vi "rsscope_core_global.vi"() -> ()   [LabVIEW 2018] (continued)
 "Instrument Options"="", "Flags"=0, "Help"="The arithmetic mode defines how the final FFT result is calculated from the individual frame results.\n\nAvailable Repeated Capabilities:\nMath: M1, M2, M3, M4, M5, M6, M7, M8\r\n\nRemote-control command(s):\nCALCulate:MATH<m>:FFT:FRAMe:ARIThmetics"}, {"Level"=3, "Class Only"=FALSE, "Identifier"="RSSCOPE_ATTR_FFT_FRAME_MAX_FRAME_COUNT", "Descriptive Name"="FFT Frame Max Frame Count", "Data Type"=0, "Command"="CALC:MATH{Math}:FFT:FRAM:MAXC", "Access"=2, "Range Table"="rsscope_rngFFTFrameCount", "Read Callback"="", "Write Callback"="", "Supported Models"="", "Instrument Options"="", "Flags"=0, "Help"="Restricts the maximum number of frames to be calculated. Due to the other parameter settings, the required number of frames may become very high, thus slowing performance. By restricting the number of frames, you can avoid performance loss without changing the other parameters.\n\nAvailable Repeated Capabilities:\nMath: M1, M2, M3, M4, M5, M6, M7, M8\r\n\nRemote-control command(s):\nCALCulate:MATH<m>:FFT:FRAMe:MAXCount"}, {"Level"=3, "Class Only"=FALSE, "Identifier"="RSSCOPE_ATTR_FFT_FRAME_COVERAGE", "Descriptive Name"="FFT Frame Coverage", "Data Type"=1, "Command"="CALC:MATH{Math}:FFT:FRAM:COV?", "Access"=0, "Range Table"="", "Read Callback"="", "Write Callback"="", "Supported Models"="", "Instrument Options"="", "Flags"=0, "Help"="Due to the restriction of the number of frames, the waveform may only be analyzed partially. This attribute queries the percentage of the trace that was analyzed, i.e. which part of the trace was included in the frame calculation.\n\nAvailable Repeated Capabilities:\nMath: M1, M2, M3, M4, M5, M6, M7, M8\r\n\nRemote-control command(s):\nCALCulate:MATH<m>:FFT:FRAMe:COVerage?"}, {"Level"=3, "Class Only"=FALSE, "Identifier"="RSSCOPE_ATTR_FFT_FRAME_OVERLAP_FACTOR", "Descriptive Name"="FFT Frame Overlap Factor", "Data Type"=0, "Command"="CALC:MATH{Math}:FFT:FRAM:OFAC", "Access"=2, "Range Table"="rsscope_rngFFTOverlapFactor", "Read Callback"="", "Write Callback"="", "Supported Models"="", "Instrument Options"="", "Flags"=0, "Help"="Defines the minimum factor by which two neighboring frames overlap. If the required number of frames to cover the input values allows for more overlap, the factor is increased.\nThe higher the overlap factor, the more frames are used. This leads to more individual results and improves detection of transient signal effects. However, it also extends the duration of the calculation.\n\nAvailable Repeated Capabilities:\nMath: M1, M2, M3, M4, M5, M6, M7, M8\r\n\nRemote-control command(s):\nCALCulate:MATH<m>:FFT:FRAMe:OFACtor"}, {"Level"=3, "Class Only"=FALSE, "Identifier"="RSSCOPE_ATTR_FFT_GATE_ENABLED", "Descriptive Name"="FFT Gate Enabled", "Data Type"=3, "Command"="CALC:MATH{Math}:FFT:GATE", "Access"=2, "Range Table"="", "Read Callback"="", "Write Callback"="", "Supported Models"="", "Instrument Options"="", "Flags"=0, "Help"="Enables FFT gating.\n\nAvailable Repeated Capabilities:\nMath: M1, M2, M3, M4, M5, M6, M7, M8\r\n\nRemote-control command(s):\nCALCulate:MATH<m>:FFT:GATE[:STATe]"}, {"Level"=3, "Class Only"=FALSE, "Identifier"="RSSCOPE_ATTR_FFT_GATE_MODE", "Descriptive Name"="FFT Gate Mode", "Data Type"=0, "Command"="CALC:MATH{Math}:FFT:GATE:MODE", "Access"=2, "Range Table"="rsscope_rngAbsRel", "Read Callback"="", "Write Callback"="", "Supported Models"="", "Instrument Options"="", "Flags"=0, "Help"="Defines whether the gate settings are configured using absolute or relative values.\n\nAvailable Repeated Capabilities:\nMath: M1, M2, M3, M4, M5, M6, M7, M8\r\n\nRemote-control command(s):\nCALCulate:MATH<m>:FFT:GATE:MODE"}, {"Level"=3, "Class Only"=FALSE, "Identifier"="RSSCOPE_ATTR_FFT_GATE_ABSOLUTE_START", "Descriptive Name"="FFT Gate Absolute Start", "Data Type"=1, "Command"="CALC:MATH{Math}:FFT:GATE:ABS:STAR", "Access"=2, "Range Table"="", "Read Callback"="", "Write Callback"="", "Supported Models"="", "Instrument Options"="", "Flags"=0, "Help"="Defines the starting value for the gate.\n\nAvailable Repeated Capabilities:\nMath: M1, M2, M3, M4, M5, M6, M7, M8\r\n\nRemote-control command(s):\nCALCulate:MATH<m>:FFT:GATE:ABSolute:STARt"}, {"Level"=3, "Class Only"=FALSE, "Identifier"="RSSCOPE_ATTR_FFT_GATE_RELATIVE_START", "Descriptive Name"="FFT Gate Relative Start", "Data Type"=1, "Command"="CALC:MATH{Math}:FFT:GATE:REL:STAR", "Access"=2, "Range Table"="RsScope_rngPercent", "Read Callback"="", "Write Callback"="", "Supported Models"="", "Instrument Options"="", "Flags"=0, "Help"="Defines the starting value for the gate in percent.\n\nAvailable Repeated Capabilities:\nMath: M1, M2, M3, M4, M5, M6, M7, M8\r\n\nRemote-control command(s):\nCALCulate:MATH<m>:FFT:GATE:RELative:STARt"}, {"Level"=3, "Class Only"=FALSE, "Identifier"="RSSCOPE_ATTR_FFT_GATE_ABSOLUTE_STOP", "Descriptive Name"="FFT Gate Absolute Stop", "Data Type"=1, "Command"="CALC:MATH{Math}:FFT:GATE:ABS:STOP", "Access"=2, "Range Table"="", "Read Callback"="", "Write Callback"="", "Supported Models"="", "Instrument Options"="", "Flags"=0, "Help"="Defines the end value for the gate.\n\nAvailable Repeated Capabilities:\nMath: M1, M2, M3, M4, M5, M6, M7, M8\r\n\nRemote-control command(s):\nCALCulate:MATH<m>:FFT:GATE:ABSolute:STOP"}, {"Level"=3, "Class Only"=FALSE, "Identifier"="RSSCOPE_ATTR_FFT_GATE_RELATIVE_STOP", "Descriptive Name"="FFT Gate Relative Stop", "Data Type"=1, "Command"="CALC:MATH{Math}:FFT:GATE:REL:STOP", "Access"=2, "Range Table"="RsScope_rngPercent", "Read Callback"="", "Write Callback"="", "Supported Models"="", "Instrument Options"="", "Flags"=0, "Help"="Defines the end value for the gate in percent.\n\nAvailable Repeated Capabilities:\nMath: M1, M2, M3, M4, M5, M6, M7, M8\r\n\nRemote-control command(s):\nCALCulate:MATH<m>:FFT:GATE:RELative:STOP"}, {"Level"=3, "Class Only"=FALSE, "Identifier"="RSSCOPE_ATTR_FFT_GATE_DISPLAY_ENABLED", "Descriptive Name"="FFT Gate Display Enabled", "Data Type"=3, "Command"="CALC:MATH{Math}:FFT:GATE:SHOW", "Access"=2, "Range Table"="", "Read Callback"="", "Write Callback"="", "Supported Models"="", "Instrument Options"="", "Flags"=0, "Help"="Indicates the gate area in the source diagram.\n\nAvailable Repeated Capabilities:\nMath: M1, M2, M3, M4, M5, M6, M7, M8\r\n\nRemote-control command(s):\nCALCulate:MATH<m>:FFT:GATE:SHOW"}, {"Level"=3, "Class Only"=FALSE, "Identifier"="RSSCOPE_ATTR_FFT_GATE_ZOOM_COUPLING_ENABLED", "Descriptive Name"="FFT Gate Zoom Coupling Enabled", "Data Type"=3, "Command"="CALC:MATH{Math}:FFT:GATE:ZCO", "Access"=2, "Range Table"="", "Read Callback"="", "Write Callback"="", "Supported Models"="", "Instrument Options"="", "Flags"=0, "Help"="If enabled, the gate area is defined identically to the zoom area for the zoom diagram.\n\nAvailable Repeated Capabilities:\nMath: M1, M2, M3, M4, M5, M6, M7, M8\r\n\nRemote-control command(s):\nCALCulate:MATH<m>:FFT:GATE:ZCOupling"}, {"Level"=3, "Class Only"=TRUE, "Identifier"="", "Descriptive Name"="Coupling", "Data Type"=0, "Command"="", "Access"=0, "Range Table"="", "Read Callback"="", "Write Callback"="", "Supported Models"="", "Instrument Options"="", "Flags"=0, "Help"="Up to four spectrum displays can be shown simultaneously, one for each math waveform. The settings for one or more spectrums can be coupled. Thus, if any FFT setting for any of the coupled spectrums are changed, they are changed for all coupled spectrums."}, {"Level"=4, "Class Only"=FALSE, "Identifier"="RSSCOPE_ATTR_FFT_COUPLED_SPECTRUM", "Descriptive Name"="FFT Coupled Spectrum", "Data Type"=3, "Command"="CALC:MATH{Math}:FFT:COUP:WITH{Math2}", "Access"=2, "Range Table"="", "Read Callback"="", "Write Callback"="", "Supported Models"="", "Instrument Options"="", "Flags"=0, "Help"="Copies the current FFT settings of the selected math waveform (m) to the other selected math waveform (m2), and couples the two waveforms. This can be repeated for all math waveforms.\n\nIf any FFT setting for any of the coupled spectrums is changed, it is changed for all coupled spectrums.\n\nAvailable Repeated Capabilities:\nMath: M1, M2, M3, M4, M5, M6, M7, M8\r\nMath2: M21, M22, M23, M24, M25, M26, M27, M28\r\n\nRemote-control command(s):\nCALCulate:MATH<m>:FFT:COUPled:WITH<m2>"}, {"Level"=3, "Class Only"=TRUE, "Identifier"="", "Descriptive Name"="Spectrum Analysis", "Data Type"=0, "Command"="", "Access"=0, "Range Table"="", "Read Callback"="", "Write Callback"="", "Supported Models"="", "Instrument Options"="", "Flags"=0, "Help"="Configures FFT spectrum analysis."}, {"Level"=4, "Class Only"=FALSE, "Identifier"="RSSCOPE_ATTR_FFT_SPECTRUM_ENABLED", "Descriptive Name"="FFT Spectrum Enabled", "Data Type"=3, "Command"="CALC:MATH{Math}:FFT:SPEC:STAT", "Access"=2, "Range Table"="", "Read Callback"="", "Write Callback"="", "Supported Models"="", "Instrument Options"="K18", "Flags"=0, "Help"="Enables the spectrogram display for a math waveform.\n\nAvailable Repeated Capabilities:\nMath: M1, M2, M3, M4, M5, M6, M7, M8\r\n\nRemote-control command(s):\nCALCulate:MATH<m>:FFT:SPECtrogram:STATe"}, {"Level"=4, "Class Only"=FALSE, "Identifier"="RSSCOPE_ATTR_FFT_SPECTRUM_COLOR_TABLE_MODE", "Descriptive Name"="FFT Spectrum Color Table Mode", "Data Type"=0, "Command"="CALC:MATH{Math}:FFT:SPEC:CMOD", "Access"=2, "Range Table"="RsScope_rngFFTSpectrumColorTableMode", "Read Callback"="", "Write Callback"="", "Supported Models"="", "Instrument Options"="K18", "Flags"=0, "Help"="Selects the color table mode for the frequency analysis display.\n\nAvailable Repeated Capabilities:\nMath: M1, M2, M3, M4, M5, M6, M7, M8\r\n\nRemote-control command(s):\nCALCulate:MATH<m>:FFT:SPECtrogram:CMODe"}, {"Level"=4, "Class Only"=TRUE, "Identifier"="", "Descriptive Name"="Time Line", "Data Type"=0, "Command"="", "Access"=0, "Range Table"="", "Read Callback"="", "Write Callback"="", "Supported Models"="", "Instrument Options"="", "Flags"=0, "Help"="A time line marks a single spectrum in the spectrogram, that is: the power vs frequency results for the data acquired at a specific time. After enabling a time line, the results for that time are displayed in the spectrum diagram."}, {"Level"=5, "Class Only"=FALSE, "Identifier"="RSSCOPE_ATTR_FFT_SPECTRUM_TIME_LINE_ENABLED", "Descriptive Name"="FFT Spectrum Time Line Enabled", "Data Type"=3, "Command"="CALC:MATH{Math}:FFT:SPEC:TIM{Timeline}:STAT", "Access"=2, "Range Table"="", "Read Callback"="", "Write Callback"="", "Supported Models"="", "Instrument Options"="K18", "Flags"=0, "Help"="Enables one of two possible time lines in a spectrogram diagram. A time line marks a single waveform in the spectrogram, that is: the power vs frequency results for the data acquired at a specific time. After enabling a time line, the results for that time are displayed in the spectrum diagram.\n\nAvailable Repeated Capabilities:\nMath: M1, M2, M3, M4, M5, M6, M7, M8\r\nTimeline: TL1, TL2\r\n\nRemote-control command(s):\nCALCulate:MATH<m>:FFT:SPECtrogram:TIMeline<n>:STATe"}, {"Level"=5, "Class Only"=FALSE, "Identifier"="RSSCOPE_ATTR_FFT_SPECTRUM_TIME_LINE_POSITION", "Descriptive Name"="FFT Spectrum Time Line Position", "Data Type"=5, "Command"="CALC:MATH{Math}:FFT:SPEC:TIM{Timeline}:POS", "Access"=2, "Range Table"="RsScope_rngFFTSpectrumTimeLinePosition", "Read Callback"="", "Write Callback"="", "Supported Models"="", "Instrument Options"="K18", "Flags"=0, "Help"="Defines the position of one of the two possible time lines in a spectrogram. The time line must be enabled first.\n\nAvailable Repeated Capabilities:\nMath: M1, M2, M3, M4, M5, M6, M7, M8\r\nTimeline: TL1, TL2\r\n\nRemote-control command(s):\nCALCulate:MATH<m>:FFT:SPECtrogram:TIMeline<n>:POSition"}, {"Level"=2, "Class Only"=TRUE, "Identifier"="", "Descriptive Name"="Waveform Data", "Data Type"=0, "Command"="", "Access"=0, "Range Table"="", "Read Callback"="", "Write Callback"="", "Supported Models"="", "Instrument Options"="", "Flags"=0, "Help"="Contains functionality for reading waveform data."}, {"Level"=3, "Class Only"=FALSE, "Identifier"="RSSCOPE_ATTR_MATH_WAVEFORM_HEADER", "Descriptive Name"="Math Waveform Header", "Data Type"=2, "Command"="CALC:MATH{Math}:DATA:HEAD?", "Access"=0, "Range Table"="", "Read Callback"="", "Write Callback"="", "Supported Models"="", "Instrument Options"="", "Flags"=0, "Help"="Returns the header of math waveform data. The header contains attributes of the waveform.\n\nAvailable Repeated Capabilities:\nMath: M1, M2, M3, M4, M5, M6, M7, M8\r\n\nRemote-control command(s):\nCALCulate:MATH<m>:DATA:HEADer?"}, {"Level"=1, "Class Only"=TRUE, "Identifier"="", "Descriptive Name"="Reference Waveforms", "Data Type"=0, "Command"="", "Access"=0, "Range Table"="", "Read Callback"="", "Write Callback"="", "Supported Models"="", "Instrument Options"="", "Flags"=0, "Help"="Contains functionality for reading and configuring reference waveforms."}, {"Level"=2, "Class Only"=FALSE, "Identifier"="RSSCOPE_ATTR_REFERENCE_WAVEFORM_HEADER", "Descriptive Name"="Reference Waveform Header", "Data Type"=2, "Command"="REFC:DATA:HEAD?", "Access"=0, "Range Table"="", "Read Callback"="", "Write Callback"="", "Supported Models"="", "Instrument Options"="", "Flags"=0, "Help"="Returns the header of reference waveform data. The header contains scaling and original attributes of the waveform.\n\nAvailable Repeated Capabilities:\nNone\n\nRemote-control command(s):\nREFCurve<m>:DATA:HEADer?"}, {"Level"=2, "Class Only"=FALSE, "Identifier"="RSSCOPE_ATTR_REFERENCE_WAVEFORM_SIGNAL_TYPE", "Descriptive Name"="Reference Waveform Signal Type", "Data Type"=0, "Command"="REFC{ReferenceWfm}:DATA:STYP?", "Access"=0, "Range Table"="RsScope_rngDataSignalType", "Read Callback"="", "Write Callback"="", "Supported Models"="", "Instrument Options"="", "Flags"=0, "Help"="Returns the signal type of the source of the reference waveform.\n\nAvailable Repeated Capabilities:\nReferenceWfm: RW1, RW2, RW3, RW4\r\n\nRemote-control command(s):\nREFCurve<m>:DATA:STYPe?"}, {"Level"=2, "Class Only"=TRUE, "Identifier"="", "Descriptive Name"="Reference", "Data Type"=0, "Command"="", "Access"=0, "Range Table"="", "Read Callback"="", "Write Callback"="", "Supported Models"="", "Instrument Options"="", "Flags"=0, "Help"="Configures the reference."}, {"Level"=3, "Class Only"=FALSE, "Identifier"="RSSCOPE_ATTR_REFERENCE_WAVEFORM_SOURCE", "Descriptive Name"="Reference Waveform Source", "Data Type"=0, "Command"="REFC{ReferenceWfm}:SOUR", "Access"=2, "Range Table"="rsscope_rngWaveformParameterReference", "Read Callback"="", "Write Callback"="", "Supported Models"="", "Instrument Options"="", "Flags"=0, "Help"="Selects the source waveform to be used as a reference.\n\nAvailable Repeated Capabilities:\nReferenceWfm: RW1, RW2, RW3, RW4\r\n\nRemote-control command(s):\nREFCurve<m>:SOURce"}, {"Level"=3, "Class Only"=FALSE, "Identifier"="RSSCOPE_ATTR_REFERENCE_WAVEFORM_DISPLAY_ENABLED", "Descriptive Name"="Reference Waveform Display Enabled", "Data Type"=3, "Command"="REFC{ReferenceWfm}:STAT", "Access"=2, "Range Table"="", "Read Callback"="", "Write Callback"="", "Supported Models"="", "Instrument Options"="", "Flags"=0, "Help"="If enabled, the reference waveform is displayed in the diagram.\n\nAvailable Repeated Capabilities:\nReferenceWfm: RW1, RW2, RW3, RW4\r\n\nRemote-control command(s):\nREFCurve<m>:STATe"}, {"Level"=3, "Class Only"=FALSE, "Identifier"="RSSCOPE_ATTR_REFERENCE_WAVEFORM_NAME", "Descriptive Name"="Reference Waveform Name", "Data Type"=2, "Command"="REFC{ReferenceWfm}:NAME", "Access"=2, "Range Table"="", "Read Callback"="", "Write Callback"="", "Supported Models"="", "Instrument Options"="", "Flags"=0, "Help"="Defines the name of the reference waveform file to be loaded, saved or deleted.\n\nAvailable Repeated Capabilities:\nReferenceWfm: RW1, RW2, RW3, RW4\r\n\nRemote-control command(s):\nREFCurve<m>:NAME"}, {"Level"=3, "Class Only"=FALSE, "Identifier"="RSSCOPE_ATTR_REFERENCE_WAVEFORM_LOAD", "Descriptive Name"="Reference Waveform Load", "Data Type"=4, "Command"="REFC{ReferenceWfm}:OPEN", "Access"=1, "Range Table"="", "Read Callback"="", "Write Callback"="", "Supported Models"="", "Instrument Options"="", "Flags"=0, "Help"="Loads the reference waveform file selected by &apos;Reference Waveform Name&apos;.\n\nAvailable Repeated Capabilities:\nReferenceWfm: RW1, RW2, RW3, RW4\r\n\nRemote-control command(s):\nREFCurve<m>:OPEN"}, {"Level"=3, "Class Only"=FALSE, "Identifier"="RSSCOPE_ATTR_REFERENCE_WAVEFORM_SAVE", "Descriptive Name"="Reference Waveform Save", "Data Type"=4, "Command"="REFC{ReferenceWfm}:SAVE", "Access"=1, "Range Table"="", "Read Callback"="", "Write Callback"="", "Supported Models"="", "Instrument Options"="", "Flags"=0, "Help"="Saves the reference waveform to the file selected by &apos;Reference Waveform Name&apos;.\n\nAvailable Repeated Capabilities:\nReferenceWfm: RW1, RW2, RW3, RW4\r\n\nRemote-control command(s):\nREFCurve<m>:SAVE"}, {"Level"=3, "Class Only"=FALSE, "Identifier"="RSSCOPE_ATTR_REFERENCE_WAVEFORM_DELETE", "Descriptive Name"="Reference Waveform Delete", "Data Type"=4, "Command"="REFC{ReferenceWfm}:DEL", "Access"=1, "Range Table"="", "Read Callback"="", "Write Callback"="", "Supported Models"="", "Instrument Options"="", "Flags"=0, "Help"="Deletes the reference waveform file selected by &apos;Reference Waveform Name&apos;.\n\nAvailable Repeated Capabilities:\nReferenceWfm: RW1, RW2, RW3, RW4\r\n\nRemote-control command(s):\nREFCurve<m>:DELete"}, {"Level"=3, "Class Only"=FALSE, "Identifier"="RSSCOPE_ATTR_REFERENCE_WAVEFORM_UPDATE", "Descriptive Name"="Reference Waveform Update", "Data Type"=4, "Command"="REFC{ReferenceWfm}:UPD", "Access"=1, "Range Table"="", "Read Callback"="", "Write Callback"="", "Supported Models"="", "Instrument Options"="", "Flags"=0, "Help"="Copies the selected source waveform with all its settings to the memory of the reference waveform\n\nAvailable Repeated Capabilities:\nReferenceWfm: RW1, RW2, RW3, RW4\r\n\nRemote-control command(s):\nREFCurve<m>:UPDate"}, {"Level"=3, "Class Only"=FALSE, "Identifier"="RSSCOPE_ATTR_REFERENCE_WAVEFORM_CLEAR", "Descriptive Name"="Reference Waveform Clear", "Data Type"=4, "Command"="REFC{ReferenceWfm}:CLE", "Access"=1, "Range Table"="", "Read Callback"="", "Write Callback"="", "Supported Models"="", "Instrument Options"="", "Flags"=0, "Help"="The selected reference waveform is no longer displayed, its memory is deleted.\n\nAvailable Repeated Capabilities:\nReferenceWfm: RW1, RW2, RW3, RW4\r\n\nRemote-control command(s):\nREFCurve<m>:CLEar"}, {"Level"=3, "Class Only"=FALSE, "Identifier"="RSSCOPE_ATTR_REFERENCE_WAVEFORM_RESTORE", "Descriptive Name"="Reference Waveform Restore", "Data Type"=4, "Command"="REFC{ReferenceWfm}:REST", "Access"=1, "Range Table"="", "Read Callback"="", "Write Callback"="", "Supported Models"="", "Instrument Options"="", "Flags"=0, "Help"="Restores the settings of the source waveform, if vertical scaling is set to &apos;Independent&apos;.\n\nAvailable Repeated Capabilities:\nReferenceWfm: RW1, RW2, RW3, RW4\r\n\nRemote-control command(s):\nREFCurve<m>:RESTore"}, {"Level"=3, "Class Only"=FALSE, "Identifier"="RSSCOPE_ATTR_REFERENCE_WAVEFORM_MULTICHANNEL_FILE_NAME", "Descriptive Name"="Reference Waveform Multichannel File Name", "Data Type"=2, "Command"="REFC:MULT:NAME", "Access"=2, "Range Table"="", "Read Callback"="", "Write Callback"="", "Supported Models"="", "Instrument Options"="", "Flags"=0, "Help"="Defines the path and the file to be imported.\n\nAvailable Repeated Capabilities:\nNone\n\nRemote-control command(s):\nREFCurve<m>:MULTichannel:NAME"}, {"Level"=3, "Class Only"=FALSE, "Identifier"="RSSCOPE_ATTR_REFERENCE_WAVEFORM_MULTICHANNEL_IMPORT", "Descriptive Name"="Reference Waveform Multichannel Import", "Data Type"=0, "Command"="REFC:MULT:IMP", "Access"=2, "Range Table"="RsScope_rngWaveformMultichannelImport", "Read Callback"="", "Write Callback"="", "Supported Models"="", "Instrument Options"="", "Flags"=0, "Help"="Assigns a waveform from the multichannel file to a reference waveform. To import all waveforms that are in the file, you must assign each waveform to another reference waveform.\n\nAvailable Repeated Capabilities:\nNone\n\nRemote-control command(s):\nREFCurve<m>:MULTichannel:IMPort"}, {"Level"=3, "Class Only"=FALSE, "Identifier"="RSSCOPE_ATTR_REFERENCE_WAVEFORM_MULTICHANNEL_OPEN", "Descriptive Name"="Reference Waveform Multichannel Open", "Data Type"=4, "Command"="REFC:MULT:OPEN", "Access"=1, "Range Table"="", "Read Callback"="", "Write Callback"="", "Supported Models"="", "Instrument Options"="", "Flags"=0, "Help"="Loads the waveform data to the reference waveforms.\n\nAvailable Repeated Capabilities:\nNone\n\nRemote-control command(s):\nREFCurve<m>:MULTichannel:OPEN"}, {"Level"=2, "Class Only"=TRUE, "Identifier"="", "Descriptive Name"="Scaling", "Data Type"=0, "Command"="", "Access"=0, "Range Table"="", "Read Callback"="", "Write Callback"="", "Supported Models"="", "Instrument Options"="", "Flags"=0, "Help"="Configures scaling of the reference waveform."}, {"Level"=3, "Class Only"=FALSE, "Identifier"="RSSCOPE_ATTR_REFERENCE_WAVEFORM_VERTICAL_COUPLING", "Descriptive Name"="Reference Waveform Vertical Coupling", "Data Type"=0, "Command"="REFC{ReferenceWfm}:VMOD", "Access"=2, "Range Table"="rsscope_rngRefWfmCoupling", "Read Callback"="", "Write Callback"="", "Supported Models"="", "Instrument Options"="", "Flags"=0, "Help"="Selects the coupling of vertical settings.\n\nAvailable Repeated Capabilities:\nReferenceWfm: RW1, RW2, RW3, RW4\r\n\nRemote-control command(s):\nREFCurve<m>:VMODe"}, {"Level"=3, "Class Only"=FALSE, "Identifier"="RSSCOPE_ATTR_REFERENCE_WAVEFORM_VERTICAL_SCALE", "Descriptive Name"="Reference Waveform Vertical Scale", "Data Type"=1, "Command"="REFC{ReferenceWfm}:SCAL", "Access"=2, "Range Table"="RsScope_rngVerticalScale", "Read Callback"="", "Write Callback"="", "Supported Models"="", "Instrument Options"="", "Flags"=0, "Help"="Sets the scale factor for the reference waveform if vertical scaling is set to &apos;Independent&apos;.\n\nAvailable Repeated Capabilities:\nReferenceWfm: RW1, RW2, RW3, RW4\r\n\nRemote-control command(s):\nREFCurve<m>:SCALe"}, {"Level"=3, "Class Only"=FALSE, "Identifier"="RSSCOPE_ATTR_REFERENCE_WAVEFORM_VERTICAL_POSITION", "Descriptive Name"="Reference Waveform Vertical Position", "Data Type"=1, "Command"="REFC{ReferenceWfm}:POS", "Access"=2, "Range Table"="RsScope_rngReferenceWaveformVerticalPosition", "Read Callback"="", "Write Callback"="", "Supported Models"="", "Instrument Options"="", "Flags"=0, "Help"="Moves the reference waveform and its horizontal axis up or down in the diagram, if vertical scaling is set to &apos;Independent&apos;.\n\nAvailable Repeated Capabilities:\nReferenceWfm: RW1, RW2, RW3, RW4\r\n\nRemote-control command(s):\nREFCurve<m>:POSition"}, {"Level"=3, "Class Only"=FALSE, "Identifier"="RSSCOPE_ATTR_REFERENCE_WAVEFORM_VERTICAL_STRETCHING_ENABLED", "Descriptive Name"="Reference Waveform Vertical Stretching Enabled", "Data Type"=3, "Command"="REFC{ReferenceWfm}:RESC:VERT:STAT", "Access"=2, "Range Table"="", "Read Callback"="", "Write Callback"="", "Supported Models"="", "Instrument Options"="", "Flags"=0, "Help"="Enables and disables the vertical stretching. Stretching changes the display of the waveform independent of the vertical scale and position.\n\nAvailable Repeated Capabilities:\nReferenceWfm: RW1, RW2, RW3, RW4\r\n\nRemote-control command(s):\nREFCurve<m>:RESCale:VERTical:STATe"}, {"Level"=3, "Class Only"=FALSE, "Identifier"="RSSCOPE_ATTR_REFERENCE_WAVEFORM_VERTICAL_OFFSET", "Descriptive Name"="Reference Waveform Vertical Offset", "Data Type"=1, "Command"="REFC{ReferenceWfm}:RESC:VERT:OFFS", "Access"=2, "Range Table"="", "Read Callback"="", "Write Callback"="", "Supported Models"="", "Instrument Options"="", "Flags"=0, "Help"="Moves the reference waveform vertically. Like vertical offset of channel waveforms, the offset of a reference waveform is subtracted from the measured value.\n\nAvailable Repeated Capabilities:\nReferenceWfm: RW1, RW2, RW3, RW4\r\n\nRemote-control command(s):\nREFCurve<m>:RESCale:VERTical:OFFSet"}, {"Level"=3, "Class Only"=FALSE, "Identifier"="RSSCOPE_ATTR_REFERENCE_WAVEFORM_VERTICAL_FACTOR", "Descriptive Name"="Reference Waveform Vertical Factor", "Data Type"=1, "Command"="REFC{ReferenceWfm}:RESC:VERT:FACT", "Access"=2, "Range Table"="rsscope_rngRefWfmFactor", "Read Callback"="", "Write Callback"="", "Supported Models"="", "Instrument Options"="", "Flags"=0, "Help"="Defines the vertical stretching factor. A factor greater than 1 stretches the waveform vertically, a factor lower than 1 compresses the curve.\n\nAvailable Repeated Capabilities:\nReferenceWfm: RW1, RW2, RW3, RW4\r\n\nRemote-control command(s):\nREFCurve<m>:RESCale:VERTical:FACTor"}, {"Level"=3, "Class Only"=FALSE, "Identifier"="RSSCOPE_ATTR_REFERENCE_WAVEFORM_VERTICAL_RESET", "Descriptive Name"="Reference Waveform Vertical Reset", "Data Type"=4, "Command"="REFC{ReferenceWfm}:TOOR", "Access"=1, "Range Table"="", "Read Callback"="", "Write Callback"="", "Supported Models"="", "Instrument Options"="", "Flags"=0, "Help"="Restores the original vertical settings of the reference waveform (vertical scale, position, and offset), if vertical scaling is set to independent (see RSSCOPE_ATTR_REFERENCE_WAVEFORM_VERTICAL_COUPLING).\n\nAvailable Repeated Capabilities:\nReferenceWfm: RW1, RW2, RW3, RW4\r\n\nRemote-control command(s):\nREFCurve<m>:TOORignal"}, {"Level"=3, "Class Only"=FALSE, "Identifier"="RSSCOPE_ATTR_REFERENCE_WAVEFORM_HORZ_COUPLING", "Descriptive Name"="Reference Waveform Horizontal Coupling", "Data Type"=0, "Command"="REFC{ReferenceWfm}:HMOD", "Access"=2, "Range Table"="rsscope_rngRefWfmHorzCoupling", "Read Callback"="", "Write Callback"="", "Supported Models"="", "Instrument Options"="", "Flags"=0, "Help"="Selects the coupling of horizontal settings.\n\nAvailable Repeated Capabilities:\nReferenceWfm: RW1, RW2, RW3, RW4\r\n\nRemote-control command(s):\nREFCurve<m>:HMODe"}, {"Level"=3, "Class Only"=FALSE, "Identifier"="RSSCOPE_ATTR_REFERENCE_WAVEFORM_HORZ_STRETCHING_ENABLED", "Descriptive Name"="Reference Waveform Horizontal Stretching Enabled", "Data Type"=3, "Command"="REFC{ReferenceWfm}:RESC:HOR:STAT", "Access"=2, "Range Table"="", "Read Callback"="", "Write Callback"="", "Supported Models"="", "Instrument Options"="", "Flags"=0, "Help"="Enables and disables the horizontal stretching. Stretching changes the display of the waveform independent of the horizontal settings of the source waveform and of the horizontal diagram settings.\n\nAvailable Repeated Capabilities:\nReferenceWfm: RW1, RW2, RW3, RW4\r\n\nRemote-control command(s):\nREFCurve<m>:RESCale:HORizontal:STATe"}, {"Level"=3, "Class Only"=FALSE, "Identifier"="RSSCOPE_ATTR_REFERENCE_WAVEFORM_HORZ_OFFSET", "Descriptive Name"="Reference Waveform Horizontal Offset", "Data Type"=1, "Command"="REFC{ReferenceWfm}:RESC:HOR:OFFS", "Access"=2, "Range Table"="", "Read Callback"="", "Write Callback"="", "Supported Models"="", "Instrument Options"="", "Flags"=0, "Help"="Moves the waveform horizontally. Positive values shift the waveform to the right, negative values shift it to the left.\n\nAvailable Repeated Capabilities:\nReferenceWfm: RW1, RW2, RW3, RW4\r\n\nRemote-control command(s):\nREFCurve<m>:RESCale:HORizontal:OFFSet"}, {"Level"=3, "Class Only"=FALSE, "Identifier"="RSSCOPE_ATTR_REFERENCE_WAVEFORM_HORZ_FACTOR", "Descriptive Name"="Reference Waveform Horizontal Factor", "Data Type"=1, "Command"="REFC{ReferenceWfm}:RESC:HOR:FACT", "Access"=2, "Range Table"="rsscope_rngRefWfmFactorHorizontal", "Read Callback"="", "Write Callback"="", "Supported Models"="", "Instrument Options"="", "Flags"=0, "Help"="A factor greater than 1 stretches the waveform horizontally, a factor lower than 1 compresses the curve.\n\nAvailable Repeated Capabilities:\nReferenceWfm: RW1, RW2, RW3, RW4\r\n\nRemote-control command(s):\nREFCurve<m>:RESCale:HORizontal:FACTor"}, {"Level"=3, "Class Only"=FALSE, "Identifier"="RSSCOPE_ATTR_REFERENCE_WAVEFORM_HORIZONTAL_POSITION", "Descriptive Name"="Reference Waveform Horizontal Position", "Data Type"=1, "Command"="REFC{ReferenceWfm}:RESC:HOR:POS", "Access"=2, "Range Table"="", "Read Callback"="", "Write Callback"="", "Supported Models"="", "Instrument Options"="", "Flags"=0, "Help"="Moves the waveform horizontally. Enter a value with a time unit suitable for the time scale of the diagram. Positive values shift the waveform to the right, negative values shift it to the left.\n\nAvailable Repeated Capabilities:\nReferenceWfm: RW1, RW2, RW3, RW4\r\n\nRemote-control command(s):\nREFCurve<m>:RESCale:HORizontal:POSition"}, {"Level"=1, "Class Only"=TRUE, "Identifier"="", "Descriptive Name"="Mask Testing", "Data Type"=0, "Command"="", "Access"=0, "Range Table"="", "Read Callback"="", "Write Callback"="", "Supported Models"="", "Instrument Options"="", "Flags"=0, "Help"="Masks are used to determine whether the signal remains within specified limits, e.g. to\nuncover signal anomalies or test compliance and stability of digital signals. The limits are\nspecified as &apos;mask&apos;, which is laid over the input signal in the display. Thus you can easily\ndetect where the signal violates the mask.\nMask testing with R&S RTO has only a minor impact on the acquisition rate, thus mask\nviolations are detected very fast and reliably.\nWith R&S RTO, you can define own masks easily. Specific actions can be executed when\nmask violations occur. For error analysis, you can stop the acquisition on a failed test and\nuse the history view to look at the previous waveforms."}, {"Level"=2, "Class Only"=FALSE, "Identifier"="RSSCOPE_ATTR_SELECTED_MASK_NAME", "Descriptive Name"="Selected Mask Name", "Data Type"=2, "Command"="", "Access"=2, "Range Table"="", "Read Callback"="", "Write Callback"="", "Supported Models"="", "Instrument Options"="", "Flags"=2, "Help"="This attribute selects the mask name used for following attributes.\n\nAvailable Repeated Capabilities:\nNone\n\nRemote-control command(s):\ncmd"}, {"Level"=2, "Class Only"=TRUE, "Identifier"="", "Descriptive Name"="Results", "Data Type"=0, "Command"="", "Access"=0, "Range Table"="", "Read Callback"="", "Write Callback"="", "Supported Models"="", "Instrument Options"="", "Flags"=0, "Help"="This class returns the test results."}, {"Level"=3, "Class Only"=FALSE, "Identifier"="RSSCOPE_ATTR_MASK_TEST_RESULT_ACQUISITION_COMPLETE", "Descriptive Name"="Mask Test Result Acquisition Complete", "Data Type"=0, "Command"="MTES:RES:COUN:WAV?", "Access"=0, "Range Table"="", "Read Callback"="rsscope_formatMaskNameInt32_ReadCallback.vi", "Write Callback"="", "Supported Models"="", "Instrument Options"="", "Flags"=0, "Help"="Returns the number of tested acquisitions.\n\nAvailable Repeated Capabilities:\nNone\n\nRemote-control command(s):\nMTESt:RESult:COUNt:WAVeforms?"}, {"Level"=3, "Class Only"=FALSE, "Identifier"="RSSCOPE_ATTR_MASK_TEST_RESULT_ACQUISITION_REMAINING", "Descriptive Name"="Mask Test Result Acquisition Remaining", "Data Type"=0, "Command"="MTES:RES:COUN:REM?", "Access"=0, "Range Table"="", "Read Callback"="rsscope_formatMaskNameInt32_ReadCallback.vi", "Write Callback"="", "Supported Models"="", "Instrument Options"="", "Flags"=0, "Help"="Returns the remaining acquisitions until &apos;Average count / Nx Single count&apos; is reached.\n\nAvailable Repeated Capabilities:\nNone\n\nRemote-control command(s):\nMTESt:RESult:COUNt:REMaining?"}, {"Level"=3, "Class Only"=FALSE, "Identifier"="RSSCOPE_ATTR_MASK_TEST_RESULT_STATE", "Descriptive Name"="Mask Test Result State", "Data Type"=0, "Command"="MTES:RES:STAT?", "Access"=0, "Range Table"="RsScope_rngMaskTestResultState", "Read Callback"="rsscope_formatMaskNameInt32_ReadCallback.vi", "Write Callback"="", "Supported Models"="", "Instrument Options"="", "Flags"=0, "Help"="Returns whether the test is running or has finished. The state is set to &apos;Finished&apos; if no acquisitions remain.\n\nAvailable Repeated Capabilities:\nNone\n\nRemote-control command(s):\nMTESt:RESult:STATe?"}, {"Level"=3, "Class Only"=FALSE, "Identifier"="RSSCOPE_ATTR_MASK_TEST_RESULT_SAMPLE_HITS", "Descriptive Name"="Mask Test Result Sample Hits", "Data Type"=0, "Command"="MTES:RES:COUN:FAIL?", "Access"=0, "Range Table"="", "Read Callback"="rsscope_formatMaskNameInt32_ReadCallback.vi", "Write Callback"="", "Supported Models"="", "Instrument Options"="", "Flags"=0, "Help"="Returns the number of sample hits that violated the mask.\n\nAvailable Repeated Capabilities:\nNone\n\nRemote-control command(s):\nMTESt:RESult:COUNt:FAILures?"}, {"Level"=3, "Class Only"=FALSE, "Identifier"="RSSCOPE_ATTR_MASK_TEST_RESULT_ACQUISITION_HITS", "Descriptive Name"="Mask Test Result Acquisition Hits", "Data Type"=0, "Command"="MTES:RES:COUN:FWAV?", "Access"=0, "Range Table"="", "Read Callback"="rsscope_formatMaskNameInt32_ReadCallback.vi", "Write Callback"="", "Supported Models"="", "Instrument Options"="", "Flags"=0, "Help"="Returns the number of acquisitions that contained at least one sample hit.\n\nAvailable Repeated Capabilities:\nNone\n\nRemote-control command(s):\nMTESt:RESult:COUNt:FWAVeforms?"}, {"Level"=3, "Class Only"=FALSE, "Identifier"="RSSCOPE_ATTR_MASK_TEST_RESULT_FAIL_RATE", "Descriptive Name"="Mask Test Result Fail Rate", "Data Type"=0, "Command"="MTES:RES:FRAT?", "Access"=0, "Range Table"="", "Read Callback"="rsscope_formatMaskNameInt32_ReadCallback.vi", "Write Callback"="", "Supported Models"="", "Instrument Options"="", "Flags"=0, "Help"="Returns the ratio of acquisition hits to the number of tested acquisitions.\n\nAvailable Repeated Capabilities:\nNone\n\nRemote-control command(s):\nMTESt:RESult:FRATe?"}, {"Level"=3, "Class Only"=FALSE, "Identifier"="RSSCOPE_ATTR_MASK_TEST_RESULT", "Descriptive Name"="Mask Test Result", "Data Type"=0, "Command"="MTES:RES?", "Access"=0, "Range Table"="RsScope_rngMaskTestResult", "Read Callback"="rsscope_formatMaskNameInt32_ReadCallback.vi", "Write Callback"="", "Supported Models"="", "Instrument Options"="", "Flags"=0, "Help"="Returns the test result.\n\nAvailable Repeated Capabilities:\nNone\n\nRemote-control command(s):\nMTESt:RESult[:RESult]?"}, {"Level"=2, "Class Only"=TRUE, "Identifier"="", "Descriptive Name"="Event Actions", "Data Type"=0, "Command"="", "Access"=0, "Range Table"="", "Read Callback"="", "Write Callback"="", "Supported Models"="", "Instrument Options"="", "Flags"=0, "Help"="This class configures what happens when the mask test has failed or when it has passed successfully. Each action can be initiated either on failure or on success."}, {"Level"=3, "Class Only"=FALSE, "Identifier"="RSSCOPE_ATTR_MASK_TEST_EVENT_BEEP", "Descriptive Name"="Mask Test Event Beep", "Data Type"=0, "Command"="MTES:ONV:BEEP", "Access"=2, "Range Table"="RsScope_rngMaskTestEventAction", "Read Callback"="rsscope_formatMaskNameInt32_ReadCallback.vi", "Write Callback"="rsscope_formatMaskNameInt32_WriteCallback.vi", "Supported Models"="", "Instrument Options"="", "Flags"=0, "Help"="Generates a beep sound for the specified event.\n\nAvailable Repeated Capabilities:\nNone\n\nRemote-control command(s):\nMTESt:ONViolation:BEEP"}, {"Level"=3, "Class Only"=FALSE, "Identifier"="RSSCOPE_ATTR_MASK_TEST_EVENT_STOP", "Descriptive Name"="Mask Test Event Stop", "Data Type"=0, "Command"="MTES:ONV:STOP", "Access"=2, "Range Table"="RsScope_rngMaskTestEventAction", "Read Callback"="rsscope_formatMaskNameInt32_ReadCallback.vi", "Write Callback"="rsscope_formatMaskNameInt32_WriteCallback.vi", "Supported Models"="", "Instrument Options"="", "Flags"=0, "Help"="Stops data acquisition for the specified event.\n\nAvailable Repeated Capabilities:\nNone\n\nRemote-control command(s):\nMTESt:ONViolation:STOP"}, {"Level"=3, "Class Only"=FALSE, "Identifier"="RSSCOPE_ATTR_MASK_TEST_EVENT_PRINT", "Descriptive Name"="Mask Test Event Print", "Data Type"=0, "Command"="MTES:ONV:PRIN", "Access"=2, "Range Table"="RsScope_rngMaskTestEventAction", "Read Callback"="rsscope_formatMaskNameInt32_ReadCallback.vi", "Write Callback"="rsscope_formatMaskNameInt32_WriteCallback.vi", "Supported Models"="", "Instrument Options"="", "Flags"=0, "Help"="Prints a screenshot including the measurement results to the printer.\n\nAvailable Repeated Capabilities:\nNone\n\nRemote-control command(s):\nMTESt:ONViolation:PRINt"}, {"Level"=3, "Class Only"=FALSE, "Identifier"="RSSCOPE_ATTR_MASK_TEST_EVENT_SAVE_WAVEFORM", "Descriptive Name"="Mask Test Event Save Waveform", "Data Type"=0, "Command"="MTES:ONV:SAV", "Access"=2, "Range Table"="RsScope_rngMaskTestEventAction", "Read Callback"="rsscope_formatMaskNameInt32_ReadCallback.vi", "Write Callback"="rsscope_formatMaskNameInt32_WriteCallback.vi", "Supported Models"="", "Instrument Options"="", "Flags"=0, "Help"="Generates a beep sound for the specified event.\n\nAvailable Repeated Capabilities:\nNone\n\nRemote-control command(s):\nMTESt:ONViolation:SAVewaveform"}, {"Level"=3, "Class Only"=FALSE, "Identifier"="RSSCOPE_ATTR_MASK_TEST_EVENT_SAVE_REPORT", "Descriptive Name"="Mask Test Event Save Report", "Data Type"=0, "Command"="MTES:ONV:REP", "Access"=2, "Range Table"="RsScope_rngMaskTestEventAction", "Read Callback"="rsscope_formatMaskNameInt32_ReadCallback.vi", "Write Callback"="rsscope_formatMaskNameInt32_WriteCallback.vi", "Supported Models"="", "Instrument Options"="", "Flags"=0, "Help"="Creates and saves a report of the current settings and results.\n\nAvailable Repeated Capabilities:\nNone\n\nRemote-control command(s):\nMTESt:ONViolation:REPort"}, {"Level"=3, "Class Only"=FALSE, "Identifier"="RSSCOPE_ATTR_MASK_TEST_EVENT_START_EXTERNAL_APPLICATION", "Descriptive Name"="Mask Test Event Start External Application", "Data Type"=0, "Command"="MTES:ONV:RUN", "Access"=2, "Range Table"="RsScope_rngMaskTestEventAction", "Read Callback"="rsscope_formatMaskNameInt32_ReadCallback.vi", "Write Callback"="rsscope_formatMaskNameInt32_WriteCallback.vi", "Supported Models"="", "Instrument Options"="", "Flags"=0, "Help"="Starts an external application.\n\nAvailable Repeated Capabilities:\nNone\n\nRemote-control command(s):\nMTESt:ONViolation:RUNexec"}, {"Level"=3, "Class Only"=FALSE, "Identifier"="RSSCOPE_ATTR_MASK_TEST_EVENT_CREATE_TRIGGER_OUT_PULSE", "Descriptive Name"="Mask Test Event Create Trigger Out Pulse", "Data Type"=0, "Command"="MTES:ONV:TRIG", "Access"=2, "Range Table"="RsScope_rngMaskTestEventAction", "Read Callback"="rsscope_formatMaskNameInt32_ReadCallback.vi", "Write Callback"="rsscope_formatMaskNameInt32_WriteCallback.vi", "Supported Models"="", "Instrument Options"="", "Flags"=0, "Help"="Creates a trigger out pulse on mask violation or successful completion of the test cycle.\n\nAvailable Repeated Capabilities:\nNone\n\nRemote-control command(s):\nMTESt:ONViolation:TRIGgerout"}, {"Level"=2, "Class Only"=TRUE, "Identifier"="", "Descriptive Name"="Test Definition", "Data Type"=0, "Command"="", "Access"=0, "Range Table"="", "Read Callback"="", "Write Callback"="", "Supported Models"="", "Instrument Options"="", "Flags"=0, "Help"="Provides all settings for the mask test itself: the waveform to be tested, pass/fail conditions, and saving/loading the mask definition."}, {"Level"=3, "Class Only"=FALSE, "Identifier"="RSSCOPE_ATTR_MASK_CREATE", "Descriptive Name"="Mask Create", "Data Type"=2, "Command"="MTES:ADD", "Access"=1, "Range Table"="", "Read Callback"="", "Write Callback"="", "Supported Models"="", "Instrument Options"="", "Flags"=0, "Help"="Creates a new mask test definition with the specified name.\n\nAvailable Repeated Capabilities:\nNone\n\nRemote-control command(s):\nMTESt:ADD"}, {"Level"=3, "Class Only"=FALSE, "Identifier"="RSSCOPE_ATTR_MASK_DELETE", "Descriptive Name"="Mask Delete", "Data Type"=2, "Command"="MTES:REM", "Access"=1, "Range Table"="", "Read Callback"="", "Write Callback"="", "Supported Models"="", "Instrument Options"="", "Flags"=0, "Help"="Deletes the mask test definition with the specified name.\n\nAvailable Repeated Capabilities:\nNone\n\nRemote-control command(s):\nMTESt:REMove"}, {"Level"=3, 
